vi "IV(H)_DC_vector_magnet_fieldsweep_BF_LD-400_K6221_K2182A_PK.vi"() -> ()   [LabVIEW 2016]
uses:
  <vilib>/Math Plots/2D Math Plots/2D Compass/2D Compass XCtrl/2D Compass.xctl
  <vilib>/Math Plots/2D Math Plots/2D Compass/2D Compass Datatype/Public/Plot Helper (Vector).vi
  Labview Drivers/Keithley 622x LV 2009/Keithley 622x.lvlib
  <vilib>/Math Plots/2D Math Plots/2D Compass/2D Compass Datatype/2D Compass Datatype.lvclass
panel:
  out "2D Compass":refnum<class "2D Plot Datatype.lvclass">[](xcontrol)
  in  "Set Compliance voltage (V)":dbl=10.0 min=0.0 step=0.1 format="%_3f"
  in  "Step 3":dbl[](array[numeric])=[1e-06, 4.9e-05, 1e-06, 4.9e-05] min=-3000.0 max=3000.0 format="%.1e"
  in  "To 3":dbl[](array[numeric])=[0.00015, 0.0, -0.00015, 0.0] min=-3000.0 max=3000.0 format="%.1e"
  in  "From 3":dbl[](array[numeric])=[0.0, 0.00015, 0.0, 0.00015] min=-3000.0 max=3000.0 format="%.1e"
  in  "wait (ms)":u32=50
  in  "Nanovoltmeter 2182a VISA":refnum<visa-resource-name>="GPIB0::7::INSTR"
  in  "Current source K6221 VISA":refnum<visa-resource-name>="GPIB0::12::INSTR"
  in  "Number Averaging":i32=1
  in  "Tab Control":enum32{"Page 1", "Page 2"}(tab)=enum."Page 2"
  out "V vs I":cluster{dbl, "Field Reading":dbl}[](graph)
  out "V vs time":cluster{dbl, "Field Reading":dbl}[](graph)
  out "Magnetic Field Vector Angle":dbl=-0.0007063202353624877 format="%#_13g"
  out "Magnetic Field Vector magnitude (T)":dbl=0.04899569500372294 format="%#_13g"
  in  "From 2":dbl[](array[numeric])=[60.0] min=-3000.0 max=3000.0 format="%#.5f"
  in  "To 2":dbl[](array[numeric])=[120.0] min=-3000.0 max=3000.0 format="%#.5g"
  in  "Step 2":dbl[](array[numeric])=[5.0] min=-3000.0 max=3000.0 format="%.3g"
  in  "Wait time after each sweep(min)":dbl=0.1 format="%#_13g"
  out "Z-axis Magnetic Field (T)":string="-0.000000604\r\n"
  in  "Y-axis Field ramp rate (T/min)":string="0.005"
  in  "Z-axis Field ramp rate (T/min)":string="0.005"
  out "Z-axis (90 deg)":dbl(slide)=-6.04e-07 scale=0.0..3.0
  out "Y-Axis (0deg)":dbl(slide)=0.048995695 scale=0.0..3.0
  out "Y-axis Magnetic Field (T)":string="0.048995695\r\n"
  in  "Magnet IP Address Z-axis":string="169.254.134.245"
  in  "Magnet IP Address Y-axis":string="169.254.212.113"
  out "Resistance (ohm)":dbl=-inf format="%#_13g"
  out "Time (s)":dbl=12035.086 format="%#_13g"
  in  "Magnetic field stabilization time (s)":dbl=2.0 format="%#_13g"
  in  "Step":dbl[](array[numeric])=[0.002] min=-3000.0 max=3000.0 format="%.4g"
  in  "To":dbl[](array[numeric])=[-0.25] min=-3000.0 max=3000.0 format="%.4f"
  in  "From":dbl[](array[numeric])=[0.25] min=-3000.0 max=3000.0 format="%.4f"
  out "Iset (A)":dbl
  out "Vmeas (V)":dbl=-1.02396105e-06
  in  "Folder":path=path "D:/Pranava/Data/PtTe2/31-05-2022/001/Round2"
  out "data":dbl[](array[numeric])=[0.04899569500372294, -0.0007063202353624877, 0.0, -1.02396105e-06, -inf, 12035.086]
  in  "File name":string="021_DevB1_DC_IV_BaseT_I_14-17_V_15-18_[250_to-250mT]_[60-120deg]_5deg_steps"
  out "File path":path=path "D:/Pranava/Data/PtTe2/31-05-2022/001/Round2/021_DevB1_DC_IV_BaseT_I_14-17_V_15-18_[250_to-250mT]_[60-120deg]_5deg_steps.dat"
  # "Z-Axis: In-plane (90 deg)\nY-axis: Out-of-plane (0 deg)"
  # "[Must be less than 0.05]"
  # ".dat"
  # "It is important that there is enough time for the magnet to cool down after each sweep (Typically 15-20 min)"
  # "Configure Field Angle (deg)"
  # "Configure Field magnitude (T)"
  # "Configure current sweeps (A)"
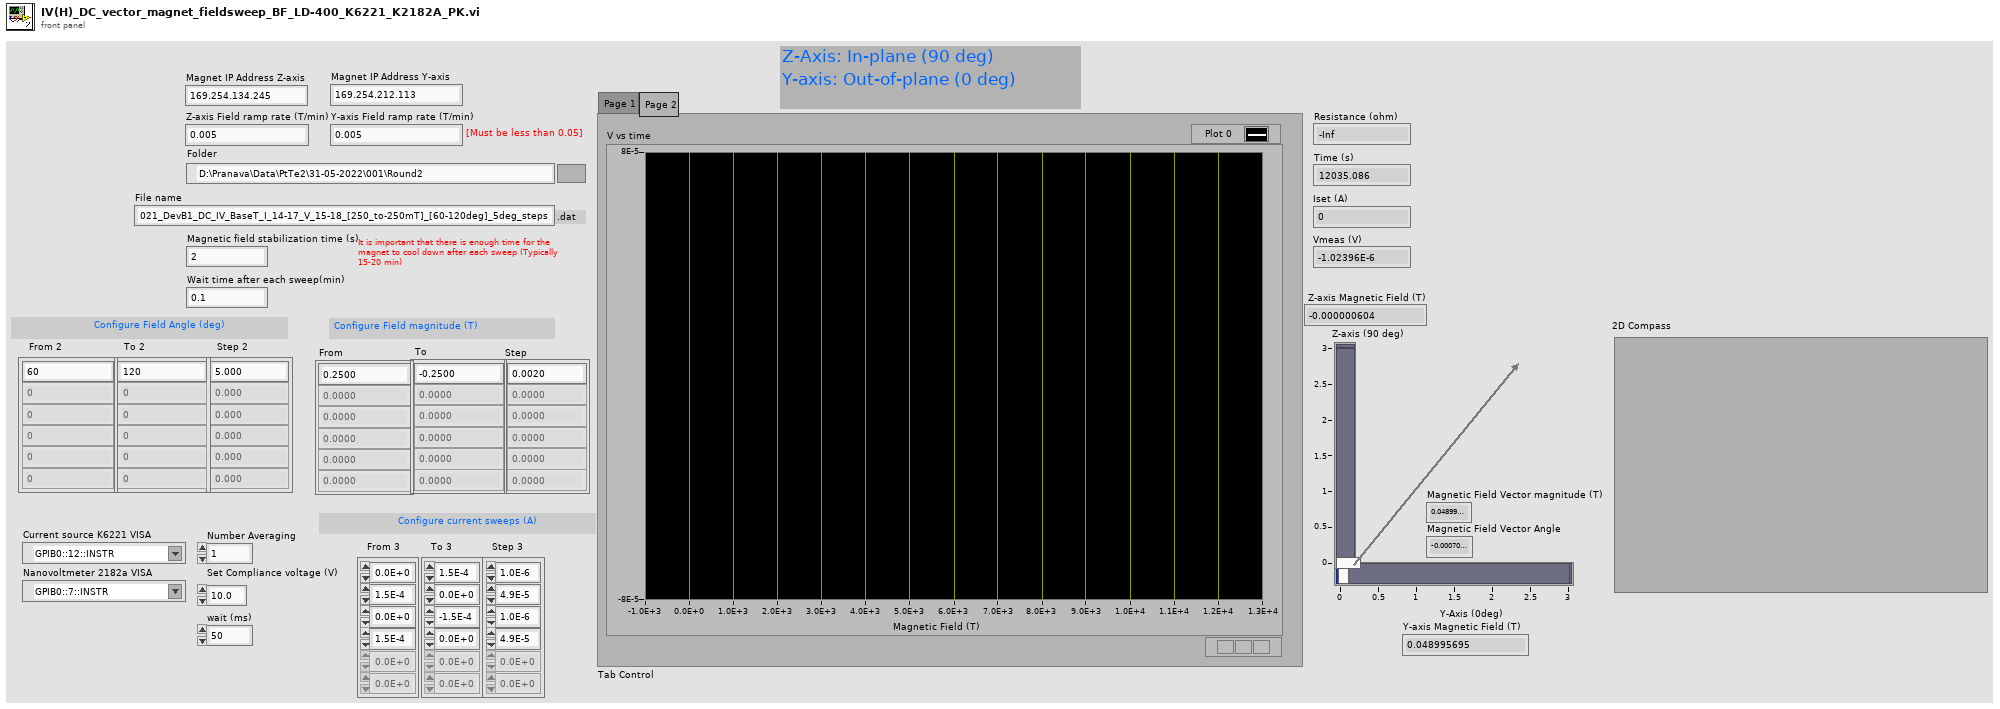
[diagram p1: front panel]
types:
  T1 = enum16{"open", "replace", "create", "open or create", "replace or create", "replace or create with confirmation"}
  T2 = typedef "Keithley 622x.lvlib/KE622x -- Current Level.ctl" = dbl
  T3 = cluster{"Average value":dbl, "Average value":dbl}
  T4 = cluster{"Average value":dbl, "Average value":dbl}[]
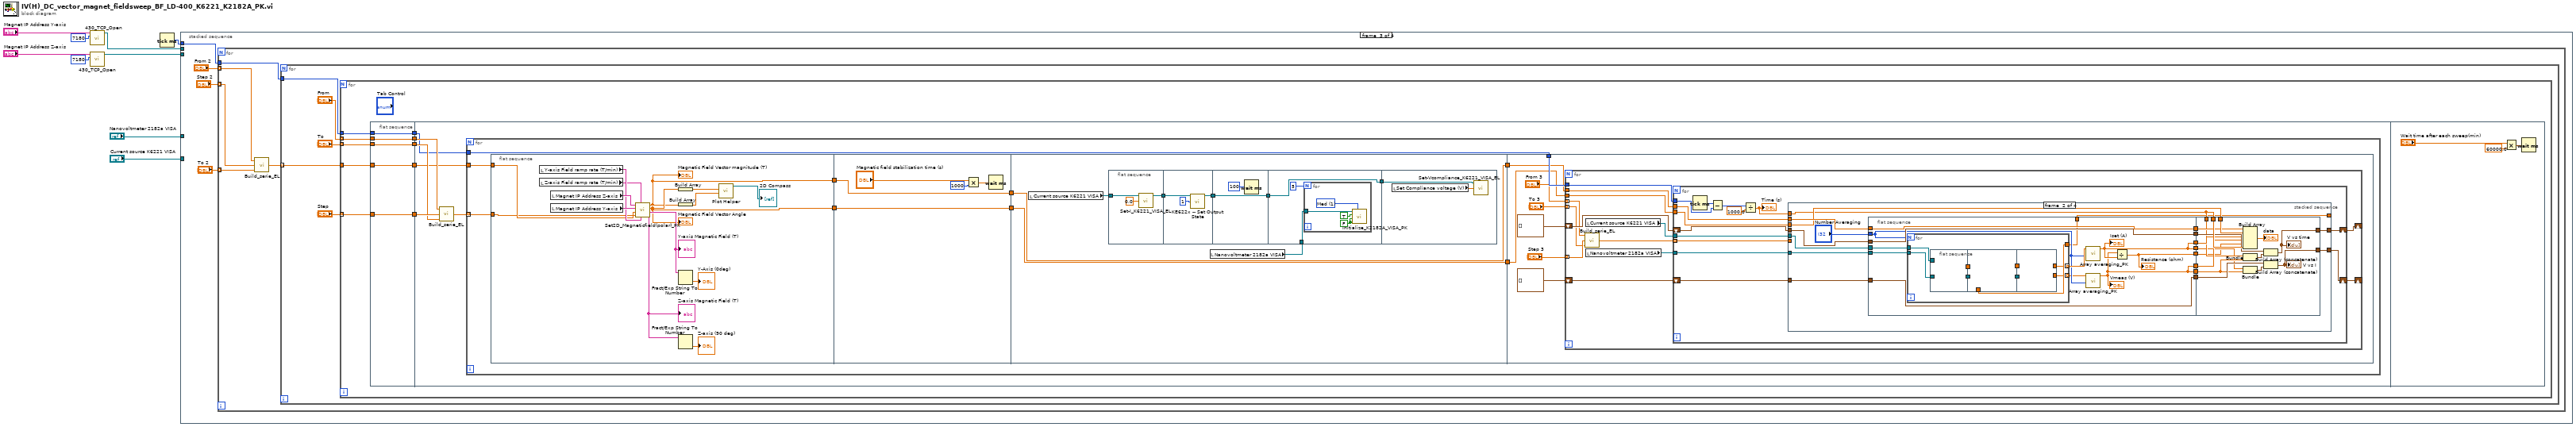
[diagram p0: block diagram]
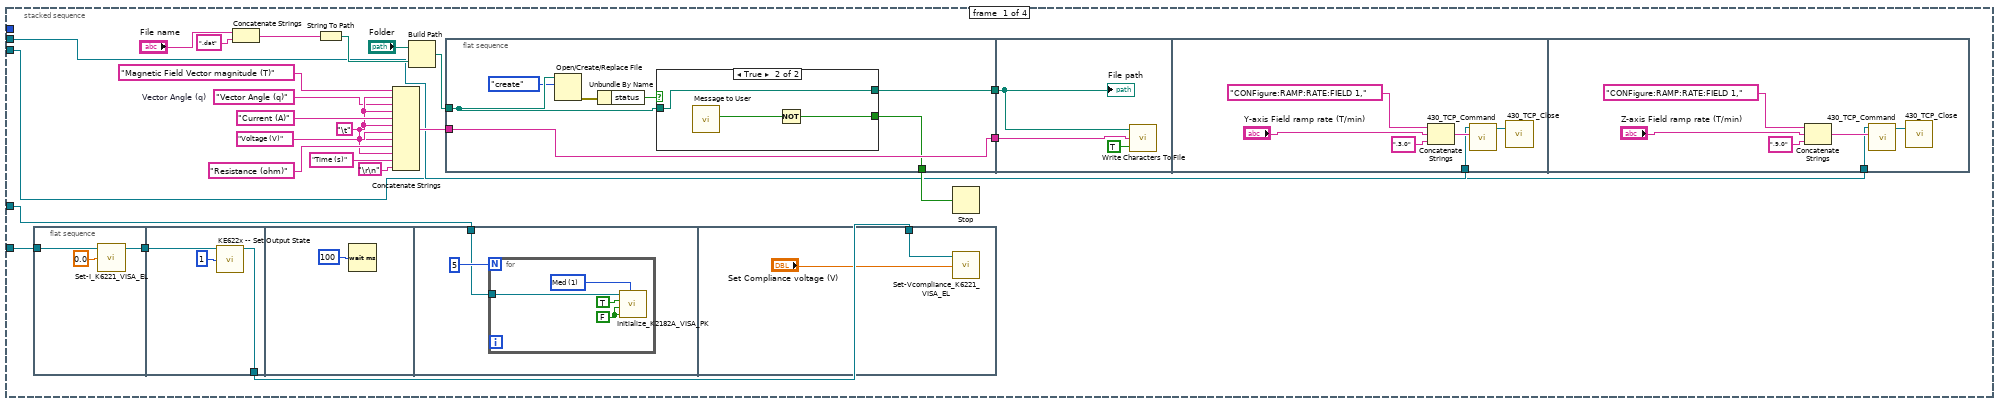
[diagram p2: hidden frame]
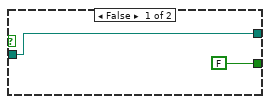
[diagram p3: hidden frame]
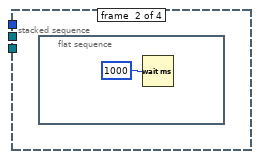
[diagram p4: hidden frame]
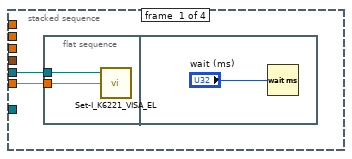
[diagram p5: hidden frame]
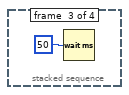
[diagram p6: hidden frame]
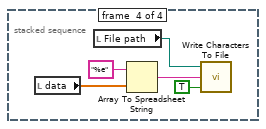
[diagram p7: hidden frame]
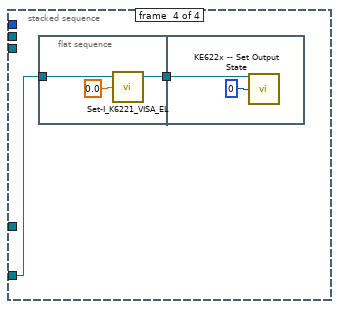
[diagram p8: hidden frame]
diagram:
  n1 = call "430_TCP_Open.vi"("IP Address"="Magnet IP Address Y-axis", "TCP Port"=7180) -> ("connection ID"=w8:refnum<k5>)  [unwired: 4 in, 2 out]
  n2 = call "430_TCP_Open.vi"("IP Address"="Magnet IP Address Z-axis", "TCP Port"=7180) -> ("connection ID"=w3:refnum<k5>)  [unwired: 4 in, 2 out]
  n3 = Tick Count (ms)() -> (millisecond timer value=w7:u32)
  n4 = stacked-sequence {
    tunnel: w8 -> [w19 _ _ _]
    tunnel: w7 -> [_ _ w80 _]
    tunnel: w3 -> [w16 _ _ _]
    tunnel: "Current source K6221 VISA" -> [w12 _ _ w280]
    tunnel: "Nanovoltmeter 2182a VISA" -> [w11 _ _ _]
    frame #0 {
      w14 = "Vector Angle (q)"  # Vector Angle (q)
      w15 = "\t"
      n5 = flat-sequence {
        tunnel: w12 -> [w36]
        tunnel: [w34] -> w13
        tunnel: w13 -> [w39]
        tunnel: [w37] -> w10
        tunnel: w11 -> [w41]
        tunnel: w10 -> [w47]
        frame #0 {
          n6 = call "Set-I_K6221_VISA_EL.vi"("Set I (A)"=0.0, "K6221 VISA"=w36) -> ("K6221 VISA out"=w34:refnum<visa-resource-name>)  [unwired: 2 in, 1 out]
        }
        frame #1 {
          n7 = call "KE622x -- Set Output State.vi"("Resource In"=w39, "Output State"=1) -> ("Resource Out (dupl)"=w37:refnum<visa-resource-name>)  [unwired: 12 in, 1 out]
        }
        frame #2 {
          n8 = Wait (ms)(milliseconds to wait=100) -> ()  [unwired: 1 out]
        }
        frame #3 {
          n9 = for {
            N: 5 ("Numeric") -> [_]
            tunnel: w41 -> [w43]
            w45 = u16 1 items=["Slow", "Med", "Fast"] ("Rate (NPLC)")
            w46 = FALSE ("Auto range?")
            n10 = call "Initialize_K2182A_VISA_PK.vi"("VISA address"=w43, "Auto range?"=TRUE, "Analog LPass\nFilter?"=w46, "DC\nFilter?"=w46, "Rate (NPLC)"=w45) -> ()  [unwired: 2 in]
          }
        }
        frame #4 {
          n11 = call "Set-Vcompliance_K6221_VISA_EL.vi"("Set Compliance voltage (V)"="Set Compliance voltage (V)", "K6221 VISA"=w47) -> ()  [unwired: 2 in, 2 out]
        }
      }
      n12 = Concatenate Strings("File name", ".dat" ("string")) -> (w29:string)
      n13 = String To Path(string=w29) -> (path=w21:path)
      n14 = Concatenate Strings("Magnetic Field Vector magnitude (T)", w15, w14, w15, "Current (A)" ("string"), w15, "Voltage (V)" ("string"), w15, "Resistance (ohm)" ("string"), w15, "Time (s)", "\r\n") -> (w30:string)
      n15 = Build Path(base path="Folder", name or relative path=w21) -> (appended path=w20:path)
      n16 = flat-sequence {
        tunnel: w20 -> [w52]
        tunnel: w30 -> [w55]
        tunnel: [w55] -> w33
        tunnel: [w54] -> w27
        tunnel: [w53] -> w32
        tunnel: w33 -> [w62]
        tunnel: w32 -> [w61]
        tunnel: w19 -> [w65]
        tunnel: w16 -> [w70]
        frame #0 {
          n17 = Open/Create/Replace File(file path (use dialog)=w52, operation (0:open)=T1."create") -> (error out=w51:errorcluster)  [unwired: 4 in, 2 out]
          n18 = Unbundle By Name(w51) -> ("status"=w49:bool)
          n19 = case shown="True" w49 {
            tunnel: [FALSE ("Yes") w59] -> w54
            tunnel: [w56 w58] -> w53
            tunnel: w52 -> [w56 w58]
            frame False {
            }
            frame True {
              n20 = call "Message to User"() -> ("Yes"=w60:bool)  [unwired: 10 in, 1 out]
              n21 = Not(x=w60) -> (.not. x?=w59:bool)
            }
          }
        }
        frame #1 {
          n22 = call <vilib>:"Write Characters To File.vi"("append to file? (new file:F)"=TRUE, "character string"=w62, "file path (dialog if empty)"=w61) -> ()  [unwired: 2 in, 1 out]
          "File path" <- w61
        }
        frame #2 {
          n23 = Concatenate Strings("CONFigure:RAMP:RATE:FIELD 1," ("String"), "Y-axis Field ramp rate (T/min)", ",3.0") -> (w66:string)
          n24 = call "430_TCP_Command.vi"("Command"=w66, "connection ID"=w65) -> ("connection ID out"=w69:refnum<k5>)  [unwired: 2 in, 2 out]
          n25 = call "430_TCP_Close.vi"("connection ID"=w69) -> ()  [unwired: 1 in, 2 out]
        }
        frame #3 {
          n26 = Concatenate Strings("CONFigure:RAMP:RATE:FIELD 1," ("String"), "Z-axis Field ramp rate (T/min)", ",9.0") -> (w72:string)
          n27 = call "430_TCP_Command.vi"("Command"=w72, "connection ID"=w70) -> ("connection ID out"=w75:refnum<k5>)  [unwired: 2 in, 2 out]
          n28 = call "430_TCP_Close.vi"("connection ID"=w75) -> ()  [unwired: 1 in, 2 out]
        }
      }
      n29 = Stop(stop? (T)=w27) -> ()
    }
    frame #1 {
      n30 = flat-sequence {
        frame #0 {
          n31 = Wait (ms)(milliseconds to wait=u32 1000) -> ()  [unwired: 1 out]
        }
      }
    }
    frame #2 {
      n32 = for {
        tunnel: w80 -> [w85]
        tunnel: "From 2" -> [w84] mode=indexing
        tunnel: "To 2" -> [w83] mode=indexing
        tunnel: "Step 2" -> [w82] mode=indexing
        n33 = call "Build_serie_EL.vi"("end value"=w83, "increment"=w82, "start value"=w84) -> ("output array"=w81:dbl[])
        n34 = for {
          tunnel: w85 -> [w87]
          tunnel: w81 -> [w86] mode=indexing
          n35 = for {
            tunnel: "From" -> [w100] mode=indexing
            tunnel: "To" -> [w98] mode=indexing
            tunnel: "Step" -> [w99] mode=indexing
            tunnel: w87 -> [w97]
            tunnel: w86 -> [w92]
            n36 = flat-sequence {
              tunnel: w97 -> [w102]
              tunnel: w98 -> [w103]
              tunnel: w99 -> [w104]
              tunnel: w100 -> [w105]
              tunnel: [w105] -> w96
              tunnel: [w104] -> w95
              tunnel: [w103] -> w94
              tunnel: [w102] -> w93
              tunnel: w92 -> [w101]
              tunnel: [w101] -> w91
              tunnel: w96 -> [w111]
              tunnel: w95 -> [w110]
              tunnel: w94 -> [w109]
              tunnel: w93 -> [w107]
              tunnel: w91 -> [w106]
              frame #0 {
              }
              frame #1 {
                n37 = call "Build_serie_EL.vi"("end value"=w109, "increment"=w110, "start value"=w111) -> ("output array"=w108:dbl[])
                n38 = for {
                  tunnel: w108 -> [w120] mode=indexing
                  tunnel: w107 -> [w119]
                  tunnel: w106 -> [w118]
                  n39 = flat-sequence {
                    tunnel: [w121] -> w117
                    tunnel: [w122] -> w116
                    tunnel: w118 -> [w127]
                    tunnel: w120 -> [w126]
                    tunnel: w117 -> [w137]
                    tunnel: [w137] -> w113
                    tunnel: [w136] -> w115
                    tunnel: w116 -> [w136]
                    tunnel: w115 -> [w148]
                    tunnel: [w148] -> w114
                    tunnel: w113 -> [w147]
                    tunnel: [w147] -> w112
                    tunnel: w114 -> [w171]
                    tunnel: w112 -> [w172]
                    tunnel: w119 -> [w173]
                    frame #0 {
                      n40 = local read "Y-axis Field ramp rate (T/min)"() -> (w133:string)
                      n41 = local read "Z-axis Field ramp rate (T/min)"() -> (w132:string)
                      n42 = local read "Magnet IP Address Z-axis"() -> (w135:string)
                      n43 = local read "Magnet IP Address Y-axis"() -> (w134:string)
                      n44 = call "Set2D_Magneticfield(polar)_PK.vi"("Y-axis Ramp Rate (T/min)"=w133, "Z-axis Ramp Rate (T/min)"=w132, "Set target vector angle (degrees)"=w127, "Set target vector magnitude (T)"=w126, "Y-Axis Magnet IP Address"=w134, "Z-Axis Magnet IP Address"=w135) -> ("Z-axis Magnetic Field (T)"=w129:string, "Y-axis Magnetic Field (T)"=w131:string, "q - Vector angle"=w122:dbl, "R - Vector field magnitude (T)"=w121:dbl)  [unwired: 2 in]
                      "Z-axis Magnetic Field (T)" <- w129
                      "Y-axis Magnetic Field (T)" <- w131
                      "Magnetic Field Vector magnitude (T)" <- w121
                      "Magnetic Field Vector Angle" <- w122
                      n45 = Build Array(w122) -> (w123:dbl[])
                      n46 = Build Array(w121) -> (w124:dbl[])
                      n47 = Fract/Exp String To Number(string=w131) -> (number=→"Y-Axis (0deg)":dbl)  [unwired: 3 in, 1 out]
                      n48 = Fract/Exp String To Number(string=w129) -> (number=→"Z-axis (90 deg)":dbl)  [unwired: 3 in, 1 out]
                      n49 = call-poly <vilib>:"Plot Helper.vi"("radius vector"=w124, "theta vector"=w123) -> ("2D Plot Class Obj Array out"=→"2D Compass":refnum<class "2D Plot Datatype.lvclass">[])  [unwired: 2 in, 7 out]
                    }
                    frame #1 {
                      n50 = Multiply(x="Magnetic field stabilization time (s)", y=1000) -> (x*y=w139:dbl)
                      n51 = Wait (ms)(milliseconds to wait=w139) -> ()  [unwired: 1 out]
                    }
                    frame #2 {
                      n52 = local read "Current source K6221 VISA"() -> (w142:refnum<visa-resource-name>)
                      n53 = flat-sequence {
                        tunnel: w142 -> [w151]
                        tunnel: [w149] -> w146
                        tunnel: w146 -> [w154]
                        tunnel: [w152] -> w145
                        tunnel: w145 -> [w155]
                        tunnel: [w155] -> w144
                        tunnel: w144 -> [w158]
                        tunnel: [w158] -> w143
                        tunnel: w141 -> [w157]
                        tunnel: w143 -> [w164]
                        frame #0 {
                          n54 = call "Set-I_K6221_VISA_EL.vi"("Set I (A)"=0.0, "K6221 VISA"=w151) -> ("K6221 VISA out"=w149:refnum<visa-resource-name>)  [unwired: 2 in, 1 out]
                        }
                        frame #1 {
                          n55 = call "KE622x -- Set Output State.vi"("Resource In"=w154, "Output State"=1) -> ("Resource Out (dupl)"=w152:refnum<visa-resource-name>)  [unwired: 12 in, 1 out]
                        }
                        frame #2 {
                          n56 = Wait (ms)(milliseconds to wait=100) -> ()  [unwired: 1 out]
                        }
                        frame #3 {
                          n57 = for {
                            N: 5 ("Numeric") -> [_]
                            tunnel: w157 -> [w160]
                            w162 = u16 1 items=["Slow", "Med", "Fast"] ("Rate (NPLC)")
                            w163 = FALSE ("Auto range?")
                            n58 = call "Initialize_K2182A_VISA_PK.vi"("VISA address"=w160, "Auto range?"=TRUE, "Analog LPass\nFilter?"=w163, "DC\nFilter?"=w163, "Rate (NPLC)"=w162) -> ()  [unwired: 2 in]
                          }
                        }
                        frame #4 {
                          n59 = local read "Set Compliance voltage (V)"() -> (w165:dbl)
                          n60 = call "Set-Vcompliance_K6221_VISA_EL.vi"("Set Compliance voltage (V)"=w165, "K6221 VISA"=w164) -> ()  [unwired: 2 in, 2 out]
                        }
                      }
                      n61 = local read "Nanovoltmeter 2182a VISA"() -> (w141:refnum<visa-resource-name>)
                    }
                    frame #3 {
                      n62 = for {
                        tunnel: w173 -> [w186]
                        tunnel: w172 -> [w184]
                        tunnel: w171 -> [w183]
                        tunnel: "From 3" -> [w178] mode=indexing
                        tunnel: "Step 3" -> [w177] mode=indexing
                        tunnel: "To 3" -> [w176] mode=indexing
                        shift-right: [w175] -> _
                        shift-left: cluster{dbl, "Field Reading":dbl}[] [] -> [w182]
                        shift-right: [w174] -> _
                        shift-left: cluster{dbl, "Field Reading":dbl}[] [] -> [w185]
                        n63 = call "Build_serie_EL.vi"("end value"=w176, "increment"=w177, "start value"=w178) -> ("output array"=w179:dbl[])
                        n64 = local read "Current source K6221 VISA"() -> (w181:refnum<visa-resource-name>)
                        n65 = local read "Nanovoltmeter 2182a VISA"() -> (w180:refnum<visa-resource-name>)
                        n66 = for {
                          tunnel: w186 -> [w200]
                          tunnel: w184 -> [w194]
                          tunnel: w183 -> [w193]
                          tunnel: w179 -> [w191] mode=indexing
                          shift-right: [w187] -> w174
                          shift-left: w185 -> [w199]
                          shift-right: [w188] -> w175
                          shift-left: w182 -> [w192]
                          tunnel: w181 -> [w190]
                          tunnel: w180 -> [w189]
                          n67 = Tick Count (ms)() -> (millisecond timer value=w196:u32)
                          n68 = Subtract(x=w196, y=w200) -> (x-y=w198:u32)
                          n69 = Divide(x=w198, y=1000.0) -> (x/y=w195:dbl)
                          "Time (s)" <- w195
                          n70 = stacked-sequence {
                            tunnel: w199 -> [_ w223 _ _]
                            tunnel: [_ w224 _ _] -> w187
                            tunnel: w195 -> [_ w211 _ _]
                            tunnel: w194 -> [_ w218 _ _]
                            tunnel: w193 -> [_ w217 _ _]
                            tunnel: [_ w216 _ _] -> w188
                            tunnel: w192 -> [_ w214 _ _]
                            tunnel: w191 -> [w202 _ _ _]
                            tunnel: [_ w208 _ _] -> _
                            tunnel: w190 -> [w201 w207 _ _]
                            tunnel: w189 -> [_ w206 _ _]
                            frame #0 {
                              n71 = flat-sequence {
                                tunnel: w202 -> [w204]
                                tunnel: w201 -> [w203]
                                frame #0 {
                                n72 = call "Set-I_K6221_VISA_EL.vi"("Set I (A)"=w204, "K6221 VISA"=w203) -> ()  [unwired: 2 in, 2 out]
                                }
                                frame #1 {
                                n73 = Wait (ms)(milliseconds to wait="wait (ms)") -> ()  [unwired: 1 out]
                                }
                              }
                            }
                            frame #1 {
                              n74 = flat-sequence {
                                tunnel: [w230] -> w222
                                tunnel: [w236] -> w221
                                tunnel: [w232] -> w220
                                tunnel: [w235] -> w219
                                tunnel: [w234] -> w215
                                tunnel: "Number Averaging" -> [w229]
                                tunnel: w214 -> [w234]
                                tunnel: w223 -> [w236]
                                tunnel: w218 -> [w235]
                                tunnel: [w230] -> w212
                                tunnel: [w232] -> w210
                                tunnel: [w233] -> w209
                                tunnel: [w227] -> w208
                                tunnel: w207 -> [w226]
                                tunnel: w206 -> [w225]
                                tunnel: w222 -> [w259]
                                tunnel: [w269] -> w224
                                tunnel: w221 -> [w268]
                                tunnel: w220 -> [w258]
                                tunnel: w219 -> [w263]
                                tunnel: w211 -> [w266]
                                tunnel: w217 -> [w265]
                                tunnel: [w261] -> w216
                                tunnel: w215 -> [w260]
                                tunnel: w212 -> [w262]
                                tunnel: w211 -> [w257]
                                tunnel: w210 -> [w256]
                                tunnel: w209 -> [w255]
                                frame #0 {
                                n75 = for {
                                N: w229 -> [_]
                                tunnel: [w238] -> w228 mode=indexing
                                tunnel: [w237] -> w231 mode=indexing
                                tunnel: w226 -> [w244]
                                tunnel: [w243] -> w227
                                tunnel: w225 -> [w245]
                                n76 = flat-sequence {
                                tunnel: w244 -> [w246]
                                tunnel: w245 -> [w248]
                                tunnel: [w248] -> w242
                                tunnel: [w247] -> w241
                                tunnel: [w250] -> w243
                                tunnel: w242 -> [w251]
                                tunnel: w241 -> [w250]
                                tunnel: [w251] -> w240
                                tunnel: [w250] -> w239
                                tunnel: [w254] -> w237
                                tunnel: w240 -> [w253]
                                tunnel: w239 -> [w254]
                                tunnel: [w252] -> w238
                                frame #0 {
                                n77 = call "KE622x -- Get Current Level.vi"("Resource In"=w246) -> ("Current Level (A)"=w247:T2)  [unwired: 12 in, 2 out]
                                }
                                frame #1 {
                                n78 = Wait (ms)(milliseconds to wait=50) -> ()  [unwired: 1 out]
                                }
                                frame #2 {
                                n79 = call "Get-V_K2182A_VISA_EL.vi"("VISA K2182A"=w253) -> ("V (V)"=w252:dbl)  [unwired: 2 in, 2 out]
                                }
                                }
                                }
                                n80 = call "Array averaging_PK.vi"("Number averaging"=w229, "numeric array"=w231) -> ("Average value"=w232:dbl)  [unwired: 9 in]
                                "Iset (A)" <- w232
                                n81 = call "Array averaging_PK.vi"("Number averaging"=w229, "numeric array"=w228) -> ("Average value"=w230:dbl)  [unwired: 9 in]
                                "Vmeas (V)" <- w230
                                n82 = Divide(x=w230, y=w232) -> (x/y=w233:dbl)
                                "Resistance (ohm)" <- w233
                                }
                                frame #1 {
                                n83 = Build Array(w263, w265, w258, w259, w255, w266) -> (→"data":dbl[])
                                n84 = Bundle(w257, "Average value"=w262) -> (w264:cluster{dbl, "Average value":dbl})  [unwired: 1 in]
                                n85 = Bundle("Average value"=w256, "Average value"=w262) -> (w267:T3)  [unwired: 1 in]
                                n86 = Build Array (concatenate)(w260, w264) -> (w261:cluster{dbl, "Average value":dbl}[])
                                "V vs time" <- w261
                                n87 = Build Array (concatenate)(w268, w267) -> (w269:T4)
                                "V vs I" <- w269
                                }
                              }
                            }
                            frame #2 {
                              n88 = Wait (ms)(milliseconds to wait=u32 50) -> ()  [unwired: 1 out]
                            }
                            frame #3 {
                              n89 = local read "data"() -> (w272:dbl[])
                              n90 = local read "File path"() -> (w274:path)
                              n91 = Array To Spreadsheet String(array=w272, 3:"%e" ("format string")) -> (spreadsheet string=w275:string)  [unwired: 1 in]
                              n92 = call <vilib>:"Write Characters To File.vi"("append to file? (new file:F)"=TRUE, "character string"=w275, "file path (dialog if empty)"=w274) -> ()  [unwired: 2 in, 1 out]
                            }
                          }
                        }
                      }
                    }
                  }
                }
              }
              frame #2 {
                n93 = Multiply(x="Wait time after each sweep(min)", y=60000.0) -> (x*y=w279:dbl)
                n94 = Wait (ms)(milliseconds to wait=w279) -> ()  [unwired: 1 out]
              }
            }
          }
        }
      }
    }
    frame #3 {
      n95 = flat-sequence {
        tunnel: w280 -> [w284]
        tunnel: [w282] -> w281
        tunnel: w281 -> [w286]
        frame #0 {
          n96 = call "Set-I_K6221_VISA_EL.vi"("Set I (A)"=0.0, "K6221 VISA"=w284) -> ("K6221 VISA out"=w282:refnum<visa-resource-name>)  [unwired: 2 in, 1 out]
        }
        frame #1 {
          n97 = call "KE622x -- Set Output State.vi"("Resource In"=w286, "Output State"=0) -> ()  [unwired: 12 in, 2 out]
        }
      }
    }
  }
